vi "Encoder2Postition_Rotation.vi"(10 "Signal from Encoder":dbl, 11 "Initial Position":dbl) -> (3 "Postion Rot":dbl)   [LabVIEW 2019]
panel:
  # "This Vi calculates from the encoder signal the absolut rotaional position in [°]."
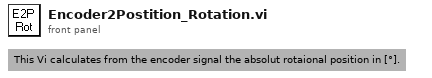
[diagram p1: front panel]
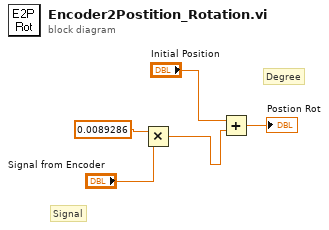
[diagram p0: block diagram]
diagram:
  # "Degree"
  # "Signal"
  n1 = Multiply(x=0.0089286, y="Signal from Encoder") -> (x*y=w1:dbl)
  n2 = Add(x="Initial Position", y=w1) -> (x+y=→"Postion Rot":dbl)
